vi "getFPGADataTelemetryEvent.vi"(11 "UserEvents in":refnum<class "UserEvents.lvclass">) -> (2 "FPGADataTelemetryEvent":refnum<user-event>, 3 "UserEvents out":refnum<class "UserEvents.lvclass">)   [LabVIEW 2016, in "UserEvents.lvclass"]
uses:
  UserEvents.lvclass
  Communicator/Topics/TelemetryFPGAData.ctl
  Types/Timestamp.ctl
  UserEvents.lvclass/UserEvents.ctl
  Types/M1M3SupportTypes.lvlib
  Communicator/M1M3Communicator.lvlib
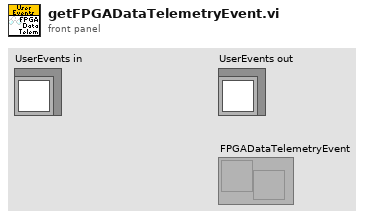
[diagram p1: front panel]
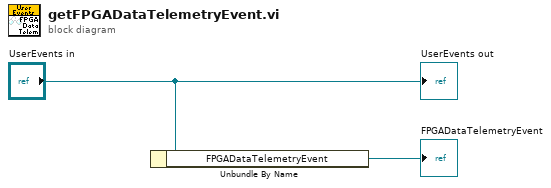
[diagram p0: block diagram]
diagram:
  n1 = Unbundle By Name("UserEvents in") -> ("FPGADataTelemetryEvent"=→"FPGADataTelemetryEvent":refnum<user-event>)
  "UserEvents out" <- "UserEvents in"
